vi "host_start_scan.vi"(8 "error in":errorcluster, 10 "initial positions":T2, 11 "index offset":T1) -> (0 "error out":errorcluster, 2 "Empty Elements Remaining":u32, 3 "out of range?":bool)   [LabVIEW 2021]
doc: "Start a scan with the initial position and index offset. This vi wait until the scan end. When input values or feedback output exceed the threshold during the scan, \"out of range\" becomes true."
uses:
  fpga/fpga_dtype_sgl_8ch.ctl
  fpga/fpga_dtype_index.ctl
  core/host_global_vars.vi
  <vilib>/Utility/error.llb/Error Cluster From Error Code.vi
  <vilib>/rvi/errors/niLvFpgaAdjustHostInterfaceError.vi
  <vilib>/rvi/interface/nirviMethod/nirviMethod.xnode
  FPGA Bitfiles/openlabspm_FPGATarget_fpgamain_eo-gUZR5D1g.lvbitx
  fpga/fpga_main.vi
  <vilib>/FPGAPlugInAG/PXIe-7856R/niLvFpga_WriteFifo_PXIe-7856R.vi
  <vilib>/rvi/errors/niLvFpgaMergeErrorWithErrorCode.vi
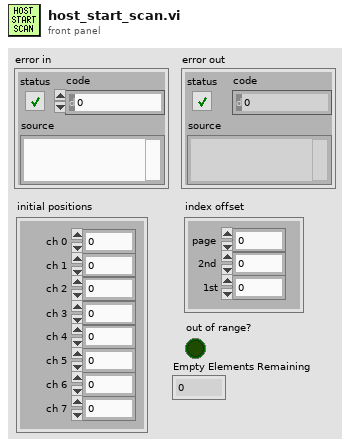
[diagram p1: front panel]
types:
  T1 = typedef "fpga_dtype_index.ctl" = cluster{"page":i16, "2nd":i16, "1st":i16}
  T2 = typedef "fpga_dtype_sgl_8ch.ctl" = cluster{"ch 0":sgl, "ch 1":sgl, "ch 2":sgl, "ch 3":sgl, "ch 4":sgl, "ch 5":sgl, "ch 6":sgl, "ch 7":sgl}
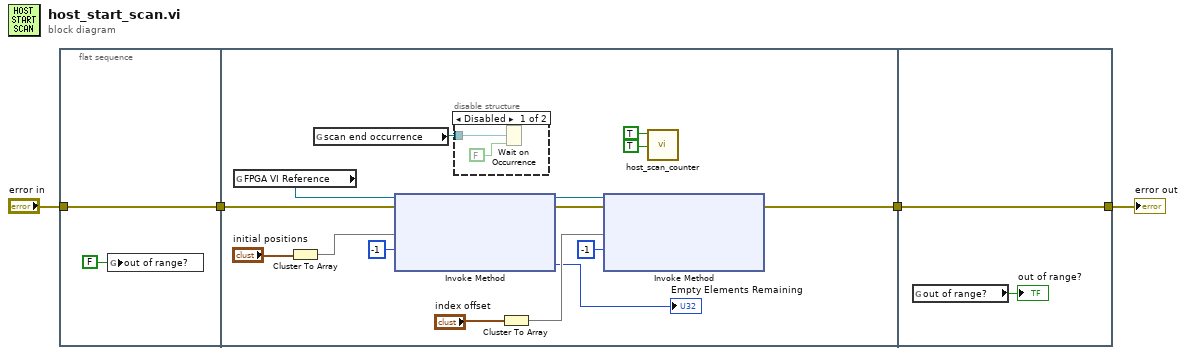
[diagram p0: block diagram]
diagram:
  n1 = flat-sequence {
    tunnel: "error in" -> [w6]
    tunnel: [w6] -> w2
    tunnel: w2 -> [w15]
    tunnel: [w12] -> w1
    tunnel: [w25] -> w3
    tunnel: w1 -> [w25]
    frame #0 {
      n2 = global write "host_global_vars.vi" "out of range?"(FALSE ("out of range?")) -> ()
    }
    frame #1 {
      n3 = global read "host_global_vars.vi" "FPGA VI Reference"() -> (w8:refnum<k20>)
      n4 = Cluster To Array(cluster="initial positions") -> (array=w16:sgl[])
      n5 = global read "host_global_vars.vi" "scan end occurrence"() -> (w21:refnum<k4>)
      n6 = xnode "Invoke Method"("FPGA VI Reference In"=w8, "error in"=w15, "Data"=w16, "Timeout (ms)"=-1) -> ("FPGA VI Reference Out"=w20:refnum<k20>, "error out"=w11:errorcluster, "Empty Elements Remaining"=→"Empty Elements Remaining":u32)
      n7 = disable-structure shown="Disabled" {
        disable-tunnel: w21 -> [w23 _]
        frame Disabled {
          n8 = Wait on Occurrence(1:FALSE ("ignore previous (T)"), 2:w23) -> ()  [unwired: 1 in, 1 out]
        }
        frame Enabled {
        }
      }
      n9 = Cluster To Array(cluster="index offset") -> (array=w13:i16[])
      n10 = xnode "Invoke Method"("FPGA VI Reference In"=w20, "error in"=w11, "Data"=w13, "Timeout (ms)"=-1) -> ("error out"=w12:errorcluster)  [unwired: 2 out]
      n11 = call "host_scan_counter.vi"("update?"=TRUE, "count up?"=TRUE) -> ()  [unwired: 9 in, 1 out]
    }
    frame #2 {
      n12 = global read "host_global_vars.vi" "out of range?"() -> (→"out of range?":bool)
    }
  }
  "error out" <- w3
